vi "Points_1_impulse.vi"(6 "Количество точек":dbl, 9 "Частота (1000 Hz)":dbl, 10 "Ширина импульса, с":dbl=1000.0, 11 "Время между импульсами, с":dbl) -> (0 "Детектор":i32[](array[numeric]), 2 "Количество точек":string caption="String", 3 "Начало второго импульса":string, 4 "Диод":i32[](array[numeric]), 5 "Оставшиеся точки":string, 7 "Начало интервала":string)   [LabVIEW 2012]
panel:
  in  "Длительность отрицательного импульса":dbl
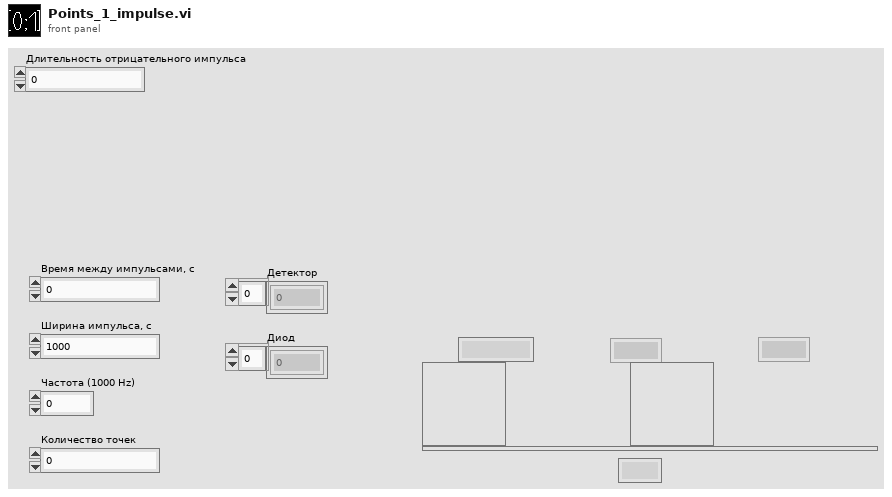
[diagram p1: front panel]
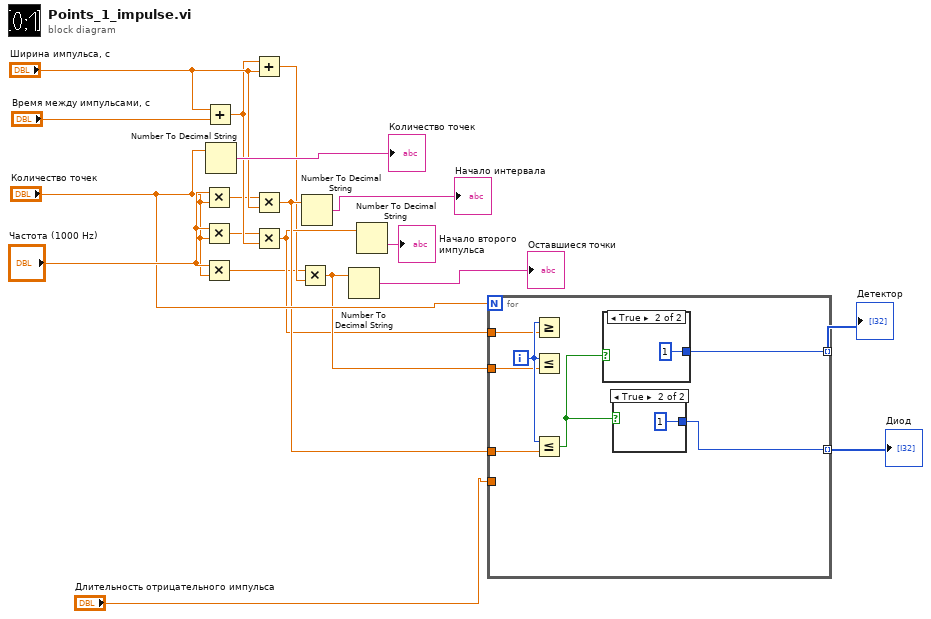
[diagram p0: block diagram]
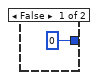
[diagram p2: hidden frame]
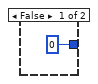
[diagram p3: hidden frame]
diagram:
  n1 = Multiply(x="Частота (1000 Hz)", y="Количество точек") -> (x*y=w4:dbl)
  n2 = Multiply(x="Частота (1000 Hz)", y="Количество точек") -> (x*y=w5:dbl)
  n3 = Multiply(x="Частота (1000 Hz)", y="Количество точек") -> (x*y=w7:dbl)
  n4 = Add(x="Ширина импульса, с", y="Время между импульсами, с") -> (x+y=w6:dbl)
  n5 = Number To Decimal String(number="Количество точек") -> (decimal integer string=→"Количество точек":string)  [unwired: 1 in]
  n6 = Add(x=w6, y="Ширина импульса, с") -> (x+y=w8:dbl)
  n7 = Multiply(x=w4, y="Ширина импульса, с") -> (x*y=w11:dbl)
  n8 = Multiply(x=w5, y=w6) -> (x*y=w9:dbl)
  n9 = Multiply(x=w7, y=w8) -> (x*y=w10:dbl)
  n10 = Number To Decimal String(number=w11) -> (decimal integer string=→"Начало интервала":string)  [unwired: 1 in]
  n11 = Number To Decimal String(number=w10) -> (decimal integer string=→"Оставшиеся точки":string)  [unwired: 1 in]
  n12 = Number To Decimal String(number=w9) -> (decimal integer string=→"Начало второго импульса":string)  [unwired: 1 in]
  n13 = for {
    N: "Количество точек" -> [_]
    tunnel: [w26] -> w2 mode=indexing
    tunnel: w11 -> [w25]
    tunnel: w9 -> [w23]
    tunnel: w10 -> [w22]
    tunnel: [w21] -> w3 mode=indexing
    tunnel: "Длительность отрицательного импульса" -> [_]
    i -> [w24]
    n14 = Greater Or Equal?(x=w24, y=w23) -> ()  [unwired: 1 out]
    n15 = Less Or Equal?(x=w24, y=w22) -> ()  [unwired: 1 out]
    n16 = Less Or Equal?(x=w24, y=w25) -> (x <= y?=w20:bool)
    n17 = case shown="True" w20 {
      tunnel: [0 1] -> w26
      frame False {
      }
      frame True {
      }
    }
    n18 = case shown="True" w20 {
      tunnel: [0 1] -> w21
      frame False {
      }
      frame True {
      }
    }
  }
  "Диод" <- w3
  "Детектор" <- w2
